vi "test_ccd_signalOut.vi"(8 "error in":errorcluster, 11 "CCD in":refnum<class "CCD.lvclass">) -> (0 "error out":errorcluster, 3 "CCD out":refnum<class "CCD.lvclass">)   [LabVIEW 2023, in "horiba.test.lvlib"]
uses:
  horiba.test.lvlib
  Classes/CCD/CCD.lvclass
  C:/Projects/Horiba/horiba-labview-sdk/Source/Classes/GenericDevice/GenericDevice.lvclass
  Classes/CCD/SignalOut.ctl
  15e7fe39-3d4f-4ccc-ae5c-22e5f2c5c50b.vi
  ea63f925-e641-4c0a-a139-6263cd42ee73.vi
  0d1025e9-6526-4eb0-922b-3647fa86469f.vi
  <vilib>/JDP Science/JSONtext/Variant to JSON Text.vi
  <vilib>/addons/_JKI Toolkits/Caraya/classes/Assert/Assert Equal Value and Type_Variant.vi
  <vilib>/JDP Science/JSONtext/LVClass Serializer/JSONtext LVClass Serializer.lvclass
  <vilib>/addons/_JKI Toolkits/Caraya/classes/Test/Test.lvclass
  <vilib>/addons/_JKI Toolkits/Caraya/classes/Assert/Assert.lvclass
  <userlib>/_OpenG.lib/lvdata/lvdata.llb/openg_variant.lvlib
panel:
  # "Connector Pane"
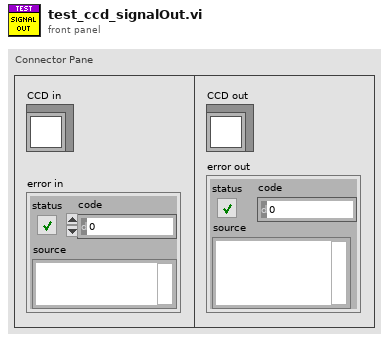
[diagram p1: front panel]
types:
  T1 = typedef "horiba.lvlib/CCD.lvclass/SignalOut.ctl" = cluster{"address":i32, "event":i32, "signalType":i32}
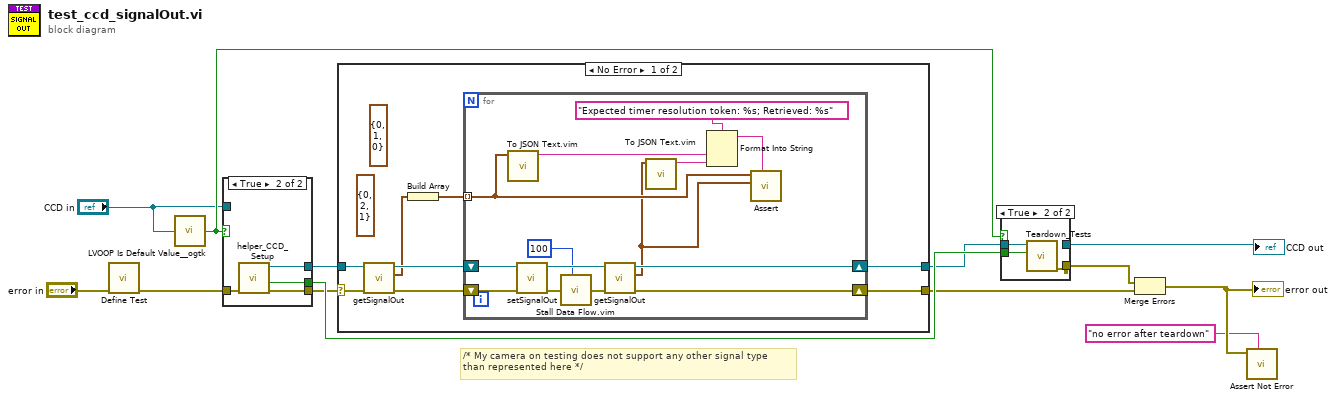
[diagram p0: block diagram]
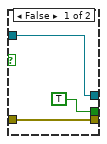
[diagram p3: hidden frame]
diagram:
  # "/* My camera on testing does not support any other signal type\nthan represented here */"
  n1 = call <vilib>:"Define Test.vi"("error in (no error)"="error in") -> ("error out"=w8:errorcluster)  [unwired: 9 in, 1 out]
  n2 = call <userlib>:"LVOOP Is Default Value__ogtk.vi"("Object"="CCD in") -> ("Is Default Value?"=w9:bool)
  n3 = case shown="True" w9 {
    tunnel: w8 -> [w15 w20]
    tunnel: [w15 w19] -> w4
    tunnel: [w16 w18] -> w6
    tunnel: [TRUE ("Module Was Already Running?") w17] -> w10
    tunnel: "CCD in" -> [w16 _]
    frame False {
    }
    frame True {
      n4 = call "helper_CCD_Setup.vi"("error in"=w20) -> ("error out"=w19:errorcluster, "Module Was Already Running?"=w17:bool, "CCD out"=w18:refnum<class "CCD.lvclass">)  [unwired: 7 in, 1 out]
    }
  }
  n5 = case shown="No Error" w4 {
    selector: w4 -> [w28 w43]
    tunnel: [w25 w44] -> w5
    tunnel: w6 -> [w27 w44]
    tunnel: [w23 w43] -> w3
    frame No Error {
      (unwired) T1 {"address"=0, "event"=2, "signalType"=1} ("Signal out")
      (unwired) T1 {"address"=0, "event"=1, "signalType"=0} ("Signal out")
      n6 = call "getSignalOut.vi"("error in (no error)"=w28, "CCD in"=w27) -> ("error out"=w24:errorcluster, "Signal out"=w21:T1, "CCD out"=w26:refnum<class "CCD.lvclass">)  [unwired: 7 in]
      n7 = Build Array(w21) -> (w22:T1[])
      n8 = for {
        shift-right: [w39] -> w25
        shift-left: w26 -> [w40]
        shift-right: [w37] -> w23
        shift-left: w24 -> [w38]
        tunnel: w22 -> [w32] mode=indexing
        n9 = call "To JSON Text.vim"("Anything"=w32) -> ("<JSON>"=w31:string)  [unwired: 9 in, 1 out]
        n10 = call "setSignalOut.vi"("error in (no error)"=w38, "CCD in"=w40) -> ("error out"=w42:errorcluster, "CCD out"=w41:refnum<class "CCD.lvclass">)  [unwired: 6 in, 2 out]
        n11 = call "Stall Data Flow.vim"("value in"=w42, "milliseconds to wait"=u32 100) -> ("value out"=w34:errorcluster)  [unwired: 1 out]
        n12 = call "getSignalOut.vi"("error in (no error)"=w34, "CCD in"=w41) -> ("error out"=w37:errorcluster, "Signal out"=w29:T1, "CCD out"=w39:refnum<class "CCD.lvclass">)  [unwired: 7 in]
        n13 = call "To JSON Text.vim"("Anything"=w29) -> ("<JSON>"=w30:string)  [unwired: 9 in, 1 out]
        n14 = Format Into String(format string="Expected timer resolution token: %s; Retrieved: %s", w31, w30) -> (resulting string=w36:string)  [unwired: 2 in, 1 out]
        n15 = call-poly <vilib>:"Assert.vi"("Label"=w36, "Y"=w29, "X"=w32) -> ()  [unwired: 7 in, 2 out]
      }
    }
    frame Error {
    }
  }
  n16 = case shown="True" w9 {
    tunnel: w5 -> [w45 w48]
    tunnel: [_ w47] -> w7
    tunnel: w10 -> [_ w46]
    tunnel: [w45 _] -> w1
    frame False {
    }
    frame True {
      n17 = call "Teardown_Tests.vi"("Module Was Already Running?"=w46, "horiba.lvlib:GenericDevice"=w48) -> ("error out"=w47:errorcluster)  [unwired: 8 in, 1 out]
    }
  }
  "CCD out" <- w1
  n18 = Merge Errors(w7, w3) -> (w12:errorcluster)
  "error out" <- w12
  n19 = call <vilib>:"Assert Not Error.vi"("Label"="no error after teardown", "Not Error?"=w12) -> ()  [unwired: 8 in, 2 out]
